vi "Global Variables.vi"() -> ()   [LabVIEW 2018]
panel:
  in  "Z dim (mm)":dbl
  in  "Sampling Frequency (Hz)":dbl=100000.0
  in  "Bleed (mm)":dbl
  in  "Max Input (V)":dbl
  in  "Min Input (V)":dbl
  in  "Step (mm)":dbl
  in  "Y dim + bleed (mm)":dbl
  in  "X dim + bleed (mm)":dbl
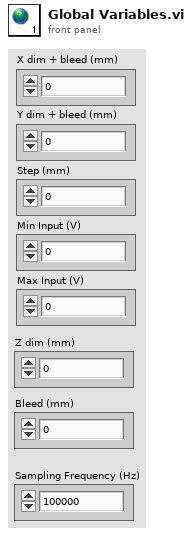
[diagram p1: front panel]
diagram:
